vi "Third SubVI.vi"(11 "logger in":refnum<class "Logger.lvclass">) -> (3 "logger out":refnum<class "Logger.lvclass">)   [LabVIEW 2018]
uses:
  src/api/logger_class/Logger.lvclass
  src/api/logger_class/Log Levels.ctl
  src/api/logger_class/Log (Parts).vi
panel:
  # "Connector Pane"
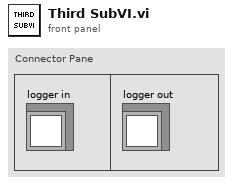
[diagram p1: front panel]
types:
  T1 = typedef "GLog.lvlib/Logger.lvclass/Log Levels.ctl" = enum16{"Trace", "Debug", "Info", "Warning", "Error", "Critical"}
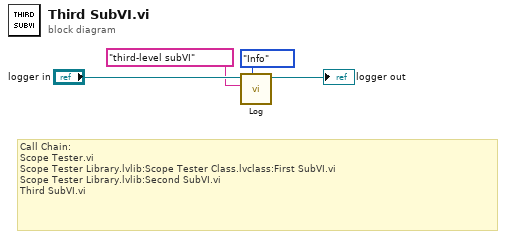
[diagram p0: block diagram]
diagram:
  # "Call Chain: \nScope Tester.vi\nScope Tester Library.lvlib:Scope Tester Class.lvclass:First SubVI.vi\nScope Tester Library.lvlib:Second SubVI.vi\nThird SubVI.vi"
  n1 = call-poly "Log.vi"("log level"=Log_Levels."Info" ("level"), "message"="third-level subVI", "logger in"="logger in") -> ("logger out"=→"logger out":refnum<class "Logger.lvclass">)  [unwired: 8 in]
